vi "FileDialog.vi"(8 "Error In":errorcluster, 11 "Path":path) -> (0 "Error Out":errorcluster, 2 "cancelled dialog?":bool caption="cancelled", 3 "Output path":path caption="selected path")   [LabVIEW 2014]
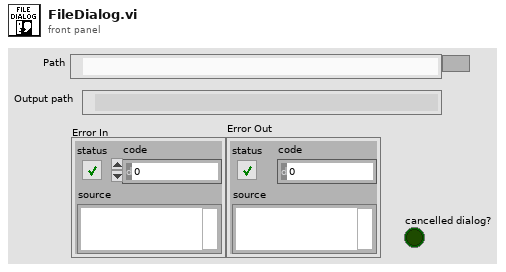
[diagram p1: front panel]
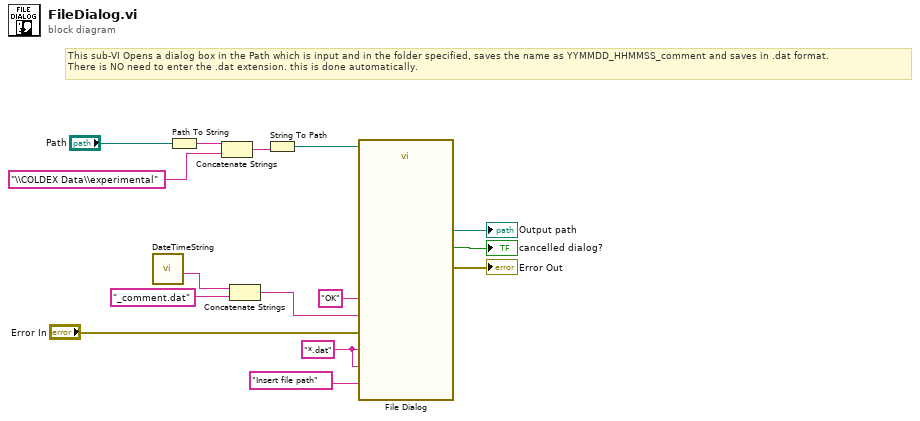
[diagram p0: block diagram]
diagram:
  w6 = "*.dat" ("pattern (all files)")
  # "This sub-VI Opens a dialog box in the Path which is input and in the folder specified, saves the name as YYMMDD_HHMMSS_comment and saves in .dat format.\nThere is NO need to enter the .dat extension. this is done automatically."
  n1 = call "DateTimeString.vi"() -> ("date/time string"=w13:string)  [unwired: 11 in]
  n2 = Path To String(path="Path") -> (string=w4:string)
  n3 = Concatenate Strings(w4, "\\COLDEX Data\\experimental" ("string")) -> (w5:string)
  n4 = Concatenate Strings(w13, "_comment.dat" ("string")) -> (w11:string)
  n5 = String To Path(string=w5) -> (path=w1:path)
  n6 = call "File Dialog"("start path"=w1, "prompt"="Insert file path", "button label"="OK", "default name"=w11, "error in"="Error In", "pattern (all files)"=w6, "pattern label"=w6) -> ("selected path"=→"Output path":path, "cancelled"=→"cancelled dialog?":bool, "error out"=→"Error Out":errorcluster)  [unwired: 5 in, 1 out]
